vi "Word_Get_Bookmarks_from_Template.vi"(7 "Template File Path":path, 11 "error in (no error)":errorcluster) -> (4 "Bookmark":string[](array[string]), 15 "error out":errorcluster)   [LabVIEW 2010, in "NI_ReportGenerationToolkit.lvlib"]
uses:
  <vilib>/addons/_office/NI_ReportGenerationToolkit.lvlib
panel:
  in  "Word._Application":refnum<k7>
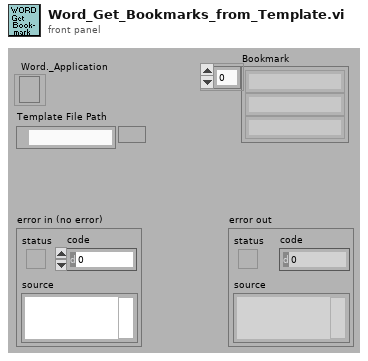
[diagram p1: front panel]
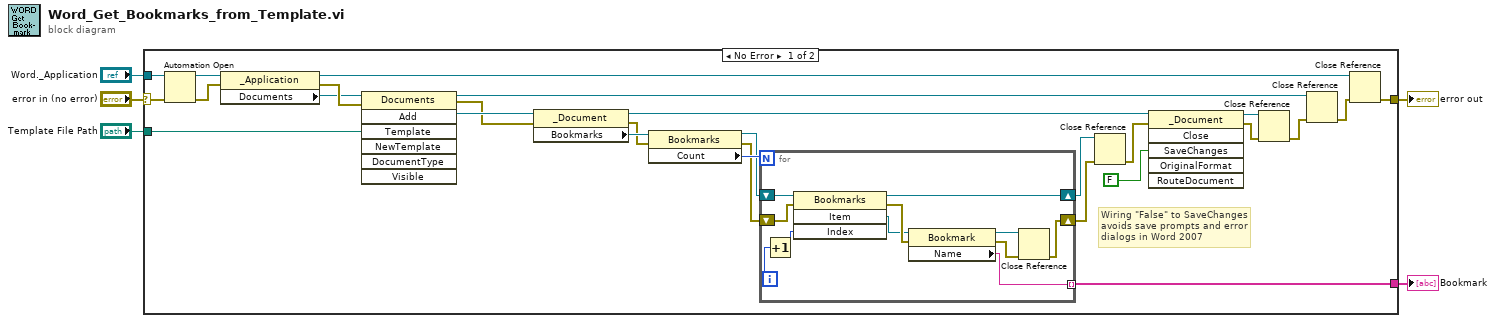
[diagram p0: block diagram]
diagram:
  n1 = case shown="No Error" "error in (no error)" {
    selector: "error in (no error)" -> [w6 w44]
    tunnel: [w32 _] -> w5
    tunnel: "Template File Path" -> [w31 _]
    tunnel: "Word._Application" -> [w15 _]
    tunnel: [w8 w44] -> w2
    frame No Error {
      # "Wiring \"False\" to SaveChanges\navoids save prompts and error\ndialogs in Word 2007"
      n2 = Automation Open(error in (no error)=w6, Automation Refnum=w15) -> (Automation Refnum=w16:refnum<k7>, error out=w17:errorcluster)  [unwired: 2 out]
      n3 = property class="_Application"(reference=w16, error in=w17) -> (reference out=w10:refnum<k7>, error out=w14:errorcluster, "Documents"=w13:refnum<k7>)
      n4 = invoke class="Documents" method="Add"(reference=w13, error in=w14, "Template"=w31) -> (reference out=w12:refnum<k7>, error out=w29:errorcluster, "Add"=w30:refnum<k7>)  [unwired: 4 in, 4 out]
      n5 = property class="_Document"(reference=w30, error in=w29) -> (reference out=w19:refnum<k7>, error out=w24:errorcluster, "Bookmarks"=w28:refnum<k7>)
      n6 = property class="Bookmarks"(reference=w28, error in=w24) -> (reference out=w25:refnum<k7>, error out=w26:errorcluster, "Count"=w27:i32)
      n7 = for {
        N: w27 -> [_]
        tunnel: [w39] -> w32 mode=indexing
        shift-right: [w36] -> w23
        shift-left: w26 -> [w38]
        shift-right: [w33] -> w22
        shift-left: w25 -> [w37]
        i -> [w42]
        n8 = Increment(x=w42) -> (x+1=w41:i32)
        n9 = invoke class="Bookmarks" method="Item"(reference=w37, error in=w38, "Index"=w41) -> (reference out=w33:refnum<k7>, error out=w43:errorcluster, "Item"=w40:refnum<k7>)  [unwired: 1 in, 1 out]
        n10 = property class="Bookmark"(reference=w40, error in=w43) -> (reference out=w34:refnum<k7>, error out=w35:errorcluster, "Name"=w39:string)
        n11 = Close Reference(reference=w34, error in (no error)=w35) -> (error out=w36:errorcluster)
      }
      n12 = Close Reference(reference=w22, error in (no error)=w23) -> (error out=w18:errorcluster)
      n13 = invoke class="_Document" method="Close"(reference=w19, error in=w18, "SaveChanges"=FALSE) -> (reference out=w20:refnum<k7>, error out=w21:errorcluster)  [unwired: 3 in, 4 out]
      n14 = Close Reference(reference=w20, error in (no error)=w21) -> (error out=w11:errorcluster)
      n15 = Close Reference(reference=w12, error in (no error)=w11) -> (error out=w9:errorcluster)
      n16 = Close Reference(reference=w10, error in (no error)=w9) -> (error out=w8:errorcluster)
    }
    frame Error {
    }
  }
  "Bookmark" <- w5
  "error out" <- w2
